vi "DB Open Reference.vi"(8 "error in (no error)":errorcluster, 11 "Database Path":path) -> (0 "error out":errorcluster, 3 "connection reference":T1)   [LabVIEW 2021, in "Database.lvlib"]
uses:
  Database.lvlib
  <vilib>/addons/database/Connection.llb/Conn ObjectReference.ctl
  <vilib>/addons/database/Connection.llb/DB Tools Open Connec (String).vi
  <vilib>/addons/database/NI_Database_API.lvlib
panel:
  in  "password":string
  in  "userID":string
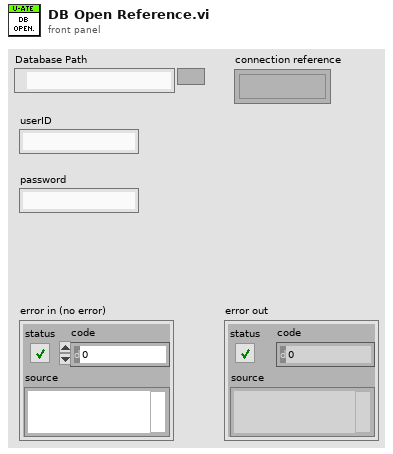
[diagram p1: front panel]
types:
  T1 = typedef "NI_Database_API.lvlib/Conn ObjectReference.ctl" = refnum<k1>
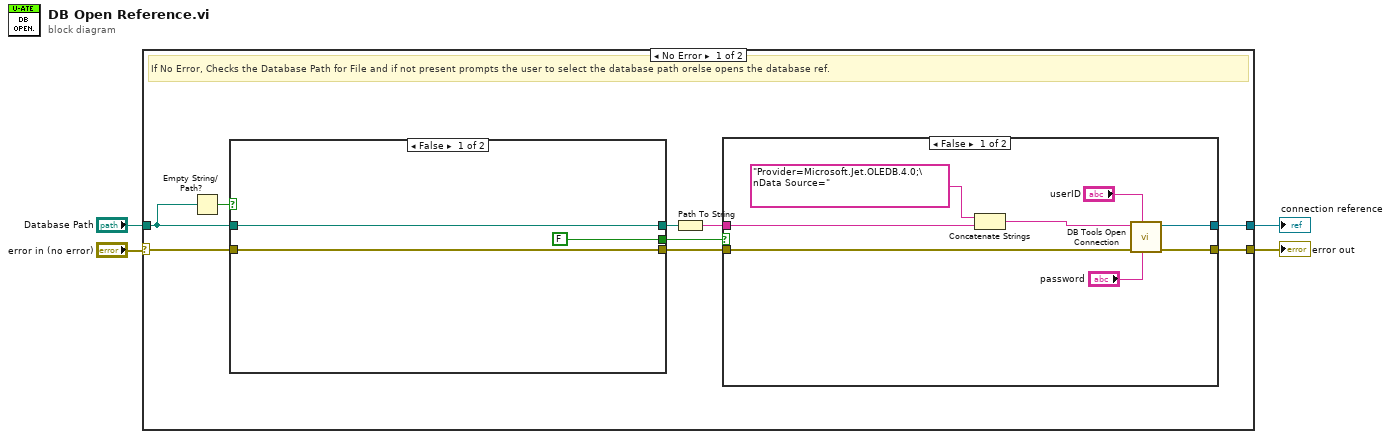
[diagram p0: block diagram]
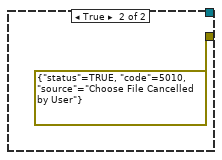
[diagram p2: hidden frame]
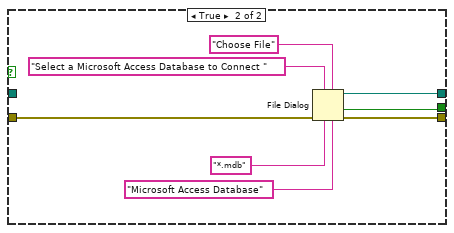
[diagram p3: hidden frame]
diagram:
  n1 = case shown="No Error" "error in (no error)" {
    selector: "error in (no error)" -> [w8 w34]
    tunnel: "Database Path" -> [w9 _]
    tunnel: [w6 _] -> w2
    tunnel: [w5 w34] -> w1
    frame No Error {
      # "If No Error, Checks the Database Path for File and if not present prompts the user to select the database path orelse opens the database ref."
      n2 = Empty String/Path?(string/path=w9) -> (empty?=w10:bool)
      n3 = case shown="False" w10 {
        tunnel: w9 -> [w25 _]
        tunnel: [w25 w29] -> w12
        tunnel: [FALSE ("cancelled") w28] -> w11
        tunnel: w8 -> [w23 w27]
        tunnel: [w23 w26] -> w7
        frame False {
        }
        frame True {
          n4 = File Dialog(4:"Microsoft Access Database" ("pattern label"), 5:"Choose File" ("button label"), 6:"*.mdb" ("pattern"), 7:"Select a Microsoft Access Database to Connect " ("prompt"), 8:w27) -> (0:w26:errorcluster, 1:w28:bool, 3:w29:path)  [unwired: 3 out]
        }
      }
      n5 = Path To String(path=w12) -> (string=w13:string)
      n6 = case shown="False" w11 {
        tunnel: w13 -> [w20 _]
        tunnel: [w17 errorcluster {"status"=TRUE, "code"=5010, "source"="Choose File Cancelled by User"} ("error out")] -> w5
        tunnel: w7 -> [w15 _]
        tunnel: [w14 _] -> w6
        frame False {
          n7 = Concatenate Strings("Provider=Microsoft.Jet.OLEDB.4.0;\nData Source=", w20) -> (w19:string)
          n8 = call-poly <vilib>:"DB Tools Open Connection.vi"("password"="password", "userID"="userID", "error in (no error)"=w15, "connection information"=w19) -> ("error out"=w17:errorcluster, "connection reference"=w14:T1)  [unwired: 1 in, 3 out]
        }
        frame True {
        }
      }
    }
    frame Error {
      # "If Error, Do Nothing"
    }
  }
  "error out" <- w1
  "connection reference" <- w2
